vi "ClusterwitharrayU32.vi"(1 "Cluster In":cluster{"Array In":u32[], "Numeric Input":u32}, 2 "Base":u32) -> (0 "Cluster Out":cluster{"Array Out":u32[], "Numeric Output":u32})   [LabVIEW 2010]
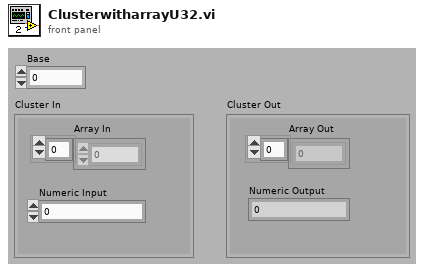
[diagram p1: front panel]
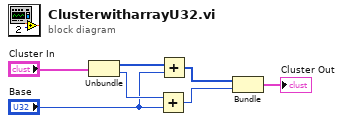
[diagram p0: block diagram]
diagram:
  n1 = Unbundle("Cluster In") -> ("Array In"=w7:u32[], "Numeric Input"=w6:u32)
  n2 = Add(x=w6, y="Base") -> (x+y=w4:u32)
  n3 = Add(x=w7, y="Base") -> (x+y=w5:u32[])
  n4 = Bundle(w5, w4) -> (→"Cluster Out":cluster{u32[], u32})  [unwired: 1 out]
